vi "parse_indep_vars.vi"(8 "error in (no error)":errorcluster, 11 "ExperimentVariables in":refnum<class "ExperimentVariables.lvclass">) -> (0 "error out":errorcluster, 3 "ExperimentVariables out":refnum<class "ExperimentVariables.lvclass">)   [LabVIEW 2013, in "ExperimentVariables.lvclass"]
uses:
  ExperimentVariables.lvclass
  ExperimentVariables.lvclass/ExperimentVariables.ctl
panel:
  out "Total Number of Data Points":i32
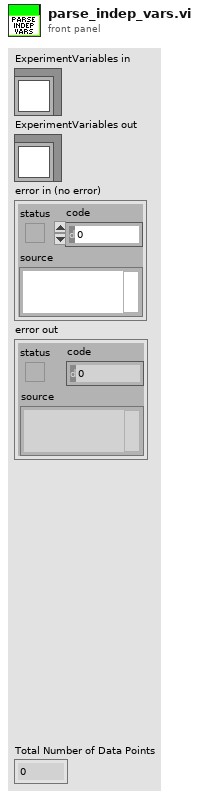
[diagram p1: front panel]
types:
  T1 = cluster{"Description":string, "Name (a,a0...a9)":string, "min":dbl, "max":dbl, "# steps":u32}[]
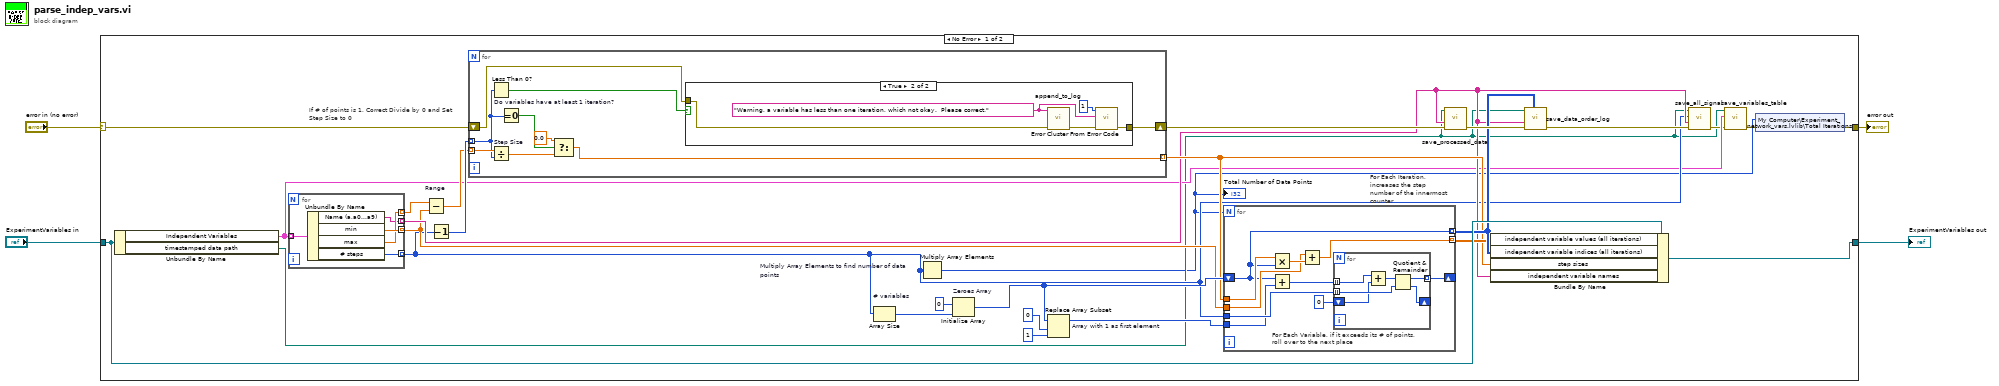
[diagram p0: block diagram]
diagram:
  n1 = case shown="No Error" "error in (no error)" {
    selector: "error in (no error)" -> [w20 w69]
    tunnel: [w5 w69] -> w3
    tunnel: [w18 w68] -> w1
    tunnel: "ExperimentVariables in" -> [w19 w68]
    frame No Error {
      n2 = Unbundle By Name(w19) -> ("Independent Variables"=w10:T1, "timestamped data path"=w8:path)
      n3 = for {
        tunnel: w10 -> [w36] mode=indexing
        tunnel: [w35] -> w13 mode=indexing
        tunnel: [w34] -> w12 mode=indexing
        tunnel: [w33] -> w11 mode=indexing
        tunnel: [w32] -> w14 mode=indexing
        n4 = Unbundle By Name(w36) -> ("Name (a,a0...a9)"=w32:string, "min"=w35:dbl, "max"=w34:dbl, "# steps"=w33:u32)
      }
      n5 = Subtract "Range"(x=w12, y=w13) -> (x-y=w30:dbl[])
      n6 = Decrement(x=w11) -> (x-1=w31:u32[])
      n7 = for "If # of points is 1, Correct Divide by 0 and Set Step Size to 0" {
        tunnel: [w60] -> w15 mode=indexing
        tunnel: w31 -> [w56] mode=indexing
        tunnel: w30 -> [w59] mode=indexing
        shift-right: [w54] -> w22
        shift-left: w20 -> [w55]
        n8 = Less Than 0? "Do variables have at least 1 iteration?"(x=w56) -> (x < 0?=w53:bool)
        n9 = Divide "Step Size"(x=w59, y=w56) -> (x/y=w58:dbl)
        n10 = Equal To 0?(x=w56) -> (x = 0?=w57:bool)
        n11 = Select(t=0.0, s=w57, f=w58) -> (s? t:f=w60:dbl)
        n12 = case shown="True" w53 {
          tunnel: w55 -> [w62 w67]
          tunnel: [w62 w65] -> w54
          frame False {
          }
          frame True {
            w64 = "Warning, a variable has less than one iteration, which not okay.  Please correct." ("string")
            n13 = call "append_to_log.vi"("error in"=w67, "string"=w64) -> ("error out"=w66:errorcluster)  [unwired: 9 in]
            n14 = call <vilib>:"Error Cluster From Error Code.vi"("error in (no error)"=w66, "error message (\"\")"=w64, "error code (0)"=1) -> ("error out"=w65:errorcluster)  [unwired: 6 in]
          }
        }
      }
      n15 = Array Size "# variables"(array=w11) -> (size(s)=w24:i32)
      n16 = Multiply Array Elements "Multiply Array Elements to find number of data points"(1:w11) -> (0:w7:u32)
      "Total Number of Data Points" <- w7
      n17 = Initialize Array "Zeroes Array"(0, w24) -> (w23:i32[])
      n18 = Replace Array Subset "Array with 1 as first element"(array=w23, new element=1 ("new element/subarray"), index=0) -> (w27:i32[])
      n19 = for "For Each Iteration, increases the step number of the innermost counter" {
        N: w7 -> [_]
        shift-right: [w37] -> _
        shift-left: w23 -> [w38]
        tunnel: w11 -> [w42]
        tunnel: w15 -> [w46]
        tunnel: [w43] -> w16 mode=indexing
        tunnel: w13 -> [w44]
        tunnel: w27 -> [w40]
        tunnel: [w38] -> w17 mode=indexing
        n20 = Multiply(x=w46, y=w38) -> (x*y=w45:dbl[])
        n21 = Add(x=w38, y=w40) -> (x+y=w39:u32[])
        n22 = Add(x=w44, y=w45) -> (x+y=w43:dbl[])
        n23 = for "For Each Variable, if it exceeds its # of points, roll over to the next place" {
          tunnel: w39 -> [w48] mode=indexing
          tunnel: w42 -> [w52] mode=indexing
          shift-right: [w51] -> _
          shift-left: 0 -> [w50]
          tunnel: [w47] -> w37 mode=indexing
          n24 = Add(x=w48, y=w50) -> (x+y=w49:u32)
          n25 = Quotient & Remainder(x=w49, y=w52) -> (x-y*floor(x/y)=w47:u32, floor(x/y)=w51:u32)
        }
      }
      n26 = call "save_processed_data.vi"("error in"=w22, "Variable Names Array"=w14, "base path"=w8) -> ("error out"=w21:errorcluster)  [unwired: 8 in]
      n27 = Bundle By Name(cluster=w19, "independent variable values (all iterations)"=w16, "independent variable indices (all iterations)"=w17, "step sizes"=w15, "independent variable names"=w14) -> (w18:refnum<class "ExperimentVariables.lvclass">)
      n28 = call "save_data_order_log.vi"("variable indices"=w17, "error in (no error)"=w21, "Variable Names Array"=w14, "file path"=w8) -> ("error out"=w26:errorcluster)  [unwired: 7 in]
      n29 = call "save_all_signal.vi"("error in (no error)"=w26, "Variable Names Array"=w14, "# of points"=w11, "file path"=w8) -> ("error out"=w9:errorcluster)  [unwired: 7 in]
      n30 = call "save_variables_table.vi"("error in"=w9, "Variable Settings.Variables"=w10, "base path"=w8) -> ("error out"=w6:errorcluster)  [unwired: 8 in]
      n31 = shared-variable "My Computer\\Experiment_network_vars.lvlib\\Total Iterations"(w7, error in=w6) -> (error out=w5:errorcluster)
    }
    frame Error {
    }
  }
  "error out" <- w3
  "ExperimentVariables out" <- w1
